vi "Test Switch when pressed.vi"(11 "Error in":errorcluster) -> (15 "Error out":errorcluster)   [LabVIEW 2020, in "Mechanical Actions Tests.lvlib"]
doc: "This VI is used to test the switch when pressed function"
uses:
  Mechanical Actions Tests.lvlib
  <vilib>/addons/_JKI Toolkits/Caraya/classes/Test Suite/Define Test Suite (JUnit Report).vi
  <vilib>/SLL Drona/APIs/Stimulus/ControlValue/SetValueAuto.vi
  <vilib>/SLL Drona/APIs/Assert/AssertControlValue/Greater.vi
  <vilib>/SLL Drona/APIs/Assert/AssertControlValue/Equal.vi
  <vilib>/SLL Drona/APIs/Stimulus/VI/CloseVI.vi
  <vilib>/Utility/error.llb/Error Cluster From Error Code.vi
  <vilib>/ErrorRing/Error Ring.xnode
  <vilib>/addons/_JKI Toolkits/Caraya/classes/Test Suite/Test Suite.lvclass
  <vilib>/addons/_JKI Toolkits/Caraya/classes/Test/Test.lvclass
  <vilib>/SLL Drona/Drona.lvlib
  <vilib>/SLL Drona/APIs/Stimulus/ControlValue/ControlValue.lvlib
  <vilib>/SLL Drona/APIs/Assert/AssertControlValue/AssertControlValue.lvlib
  <vilib>/Wiresmith Technology/G CLI/CLI Class/CLI.lvclass
  <vilib>/SLL Drona/APIs/Stimulus/VI/VI.lvlib
panel:
  # "SWITCH WHEN PRESSED TEST"
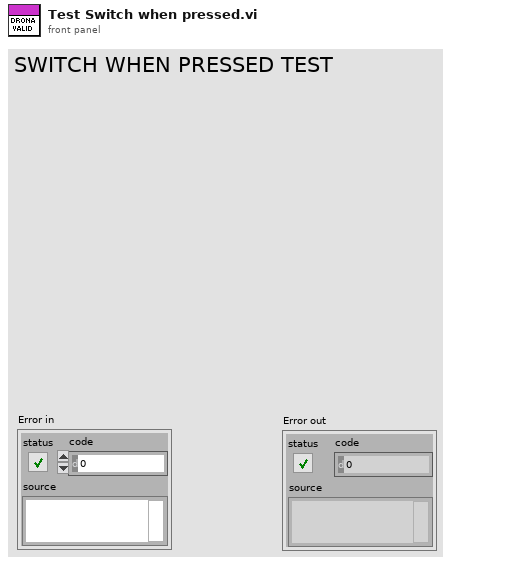
[diagram p1: front panel]
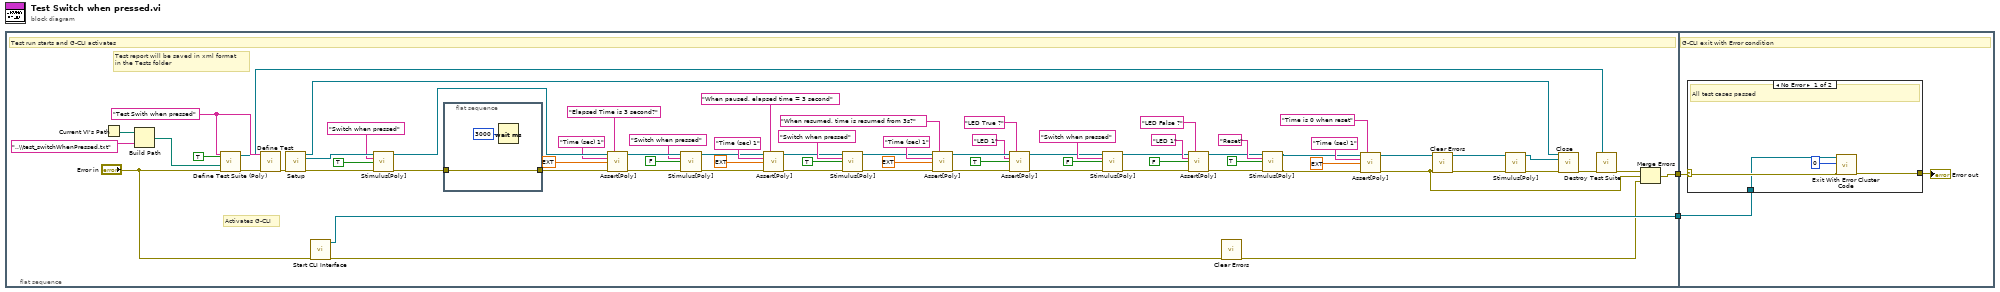
[diagram p0: block diagram]
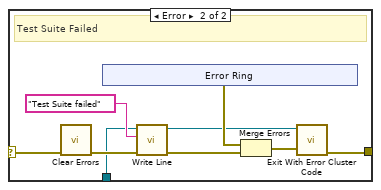
[diagram p2: hidden frame]
diagram:
  n1 = flat-sequence {
    tunnel: [w8] -> w2
    tunnel: [w6] -> w1
    tunnel: w2 -> [w78]
    tunnel: w1 -> [w77]
    frame #0 {
      w17 = "Test Swith when pressed" ("Label (VI Title)")
      # "Activates G-CLI"
      # "Test report will be saved in xml format\nin the Tests folder"
      # "Test run starts and G-CLI activates"
      n2 = Current VI's Path() -> (path=w15:path)
      n3 = Build Path(base path=w15, name or relative path="..\\test_switchWhenPressed.txt") -> (appended path=w13:path)
      n4 = call-poly <vilib>:"Define Test Suite (Poly).vi"("error in (no error)"="Error in", "Report Path"=w13, "Interactive"=TRUE, "Label (VI Title)"=w17) -> ("error out"=w18:errorcluster, "Test Suite"=w5:refnum<class "Test Suite.lvclass">)  [unwired: 5 in, 1 out]
      n5 = call <vilib>:"Define Test.vi"("error in (no error)"=w18, "Label (VI Title)"=w17) -> ("error out"=w74:errorcluster)  [unwired: 8 in, 1 out]
      n6 = call <vilib>:"Setup.vi"("error in"=w74) -> ("Application Ref"=w40:refnum<vi>, "VI Reference Out"=w72:refnum<vi>, "error out"=w73:errorcluster)  [unwired: 12 in]
      n7 = call <vilib>:"Start CLI Interface.vi"("error in (no error)"="Error in") -> ("error out"=w9:errorcluster, "CLI out"=w8:refnum<class "CLI.lvclass">)  [unwired: 7 in, 2 out]
      n8 = call-poly <vilib>:"Stimulus[Poly].vi"("VI Reference In"=w72, "Control Path"="Switch when pressed", "Value (Signaling)"=TRUE, "error in"=w73) -> ("VI Reference Out"=w67:refnum<vi>, "error out"=w69:errorcluster)  [unwired: 10 in]
      n9 = flat-sequence {
        tunnel: w69 -> [w76]
        tunnel: [w76] -> w68
        frame #0 {
          n10 = Wait (ms)(milliseconds to wait=u32 3000) -> ()  [unwired: 1 out]
        }
      }
      n11 = call-poly <vilib>:"Assert[Poly].vi"("VI Reference In"=w67, "Test Label"="Elapsed Time is 3 second?" ("Label"), "Control Path"="Time (sec) 1", "Control Value"=ext 3.0, "Error In"=w68) -> ("VI Reference Out"=w63:refnum<vi>, "Error Out"=w64:errorcluster)  [unwired: 9 in]
      n12 = call-poly <vilib>:"Stimulus[Poly].vi"("VI Reference In"=w63, "Control Path"="Switch when pressed", "Value (Signaling)"=FALSE, "error in"=w64) -> ("VI Reference Out"=w58:refnum<vi>, "error out"=w59:errorcluster)  [unwired: 10 in]
      n13 = call-poly <vilib>:"Assert[Poly].vi"("VI Reference In"=w58, "Test Label"="When paused, elapsed time = 3 second" ("Label"), "Control Path"="Time (sec) 1", "Control Value"=ext 3.0, "Error In"=w59) -> ("VI Reference Out"=w51:refnum<vi>, "Error Out"=w52:errorcluster)  [unwired: 9 in]
      n14 = call-poly <vilib>:"Stimulus[Poly].vi"("VI Reference In"=w51, "Control Path"="Switch when pressed", "Value (Signaling)"=TRUE, "error in"=w52) -> ("VI Reference Out"=w47:refnum<vi>, "error out"=w48:errorcluster)  [unwired: 10 in]
      n15 = call-poly <vilib>:"Assert[Poly].vi"("VI Reference In"=w47, "Test Label"="When resumed, time is resumed from 3s?" ("Label"), "Control Path"="Time (sec) 1", "Control Value"=ext 3.0, "Error In"=w48) -> ("VI Reference Out"=w36:refnum<vi>, "Error Out"=w33:errorcluster)  [unwired: 9 in]
      n16 = call-poly <vilib>:"Assert[Poly].vi"("VI Reference In"=w36, "Test Label"="LED True ?" ("Label"), "Control Path"="LED 1", "Control Value"=TRUE, "Error In"=w33) -> ("VI Reference Out"=w31:refnum<vi>, "Error Out"=w32:errorcluster)  [unwired: 9 in]
      n17 = call-poly <vilib>:"Stimulus[Poly].vi"("VI Reference In"=w31, "Control Path"="Switch when pressed", "Value (Signaling)"=FALSE, "error in"=w32) -> ("VI Reference Out"=w25:refnum<vi>, "error out"=w26:errorcluster)  [unwired: 10 in]
      n18 = call-poly <vilib>:"Assert[Poly].vi"("VI Reference In"=w25, "Test Label"="LED False ?" ("Label"), "Control Path"="LED 1", "Control Value"=FALSE, "Error In"=w26) -> ("VI Reference Out"=w24:refnum<vi>, "Error Out"=w23:errorcluster)  [unwired: 9 in]
      n19 = call <vilib>:"Clear Errors.vi"("error in (no error)"=w9) -> ("error out"=w7:errorcluster)  [unwired: 5 in, 1 out]
      n20 = call-poly <vilib>:"Stimulus[Poly].vi"("VI Reference In"=w24, "Control Path"="Reset", "Value (Signaling)"=TRUE, "error in"=w23) -> ("VI Reference Out"=w43:refnum<vi>, "error out"=w44:errorcluster)  [unwired: 10 in]
      n21 = call-poly <vilib>:"Assert[Poly].vi"("VI Reference In"=w43, "Test Label"="Time is 0 when reset" ("Label"), "Control Path"="Time (sec) 1", "Control Value"=ext 0.0, "Error In"=w44) -> ("VI Reference Out"=w21:refnum<vi>, "Error Out"=w3:errorcluster)  [unwired: 9 in]
      n22 = call <vilib>:"Clear Errors.vi"("error in (no error)"=w3) -> ("error out"=w4:errorcluster)  [unwired: 5 in, 1 out]
      n23 = call-poly <vilib>:"Stimulus[Poly].vi"("VI Reference In"=w21, "error in"=w4) -> ("VI Reference Out"=w20:refnum<vi>, "error out"=w19:errorcluster)  [unwired: 12 in]
      n24 = call <vilib>:"Close.vi"("Application Ref"=w40, "VI Reference"=w20, "error in"=w19) -> ("error out"=w11:errorcluster)  [unwired: 12 in]
      n25 = call-dynamic "Destroy Test Suite.vi"("error in (no error)"=w11, "Test Suite in"=w5) -> ("error out"=w10:errorcluster)  [unwired: 8 in, 1 out]
      n26 = Merge Errors(w10, w3, w7) -> (w6:errorcluster)
    }
    frame #1 {
      # "G-CLI exit with Error condition"
      n27 = case shown="No Error" w77 {
        selector: w77 -> [w83 w90]
        tunnel: [w82 w92] -> w79
        tunnel: w78 -> [w80 w85]
        frame No Error {
          # "All test cases passed"
          n28 = call <vilib>:"Exit With Error Cluster Code.vi"("error in (no error)"=w83, "No Error Code (0)"=0, "CLI in"=w80) -> ("error out"=w82:errorcluster)  [unwired: 8 in]
        }
        frame Error {
          # "Test Suite Failed"
          n29 = call <vilib>:"Clear Errors.vi"("error in (no error)"=w90) -> ("error out"=w89:errorcluster)  [unwired: 5 in, 1 out]
          n30 = xnode "Error Ring"() -> ("error out"=w87:errorcluster)
          n31 = call <vilib>:"Write Line.vi"("error in (no error)"=w89, "Text to Write"="Test Suite failed", "CLI in"=w85) -> ("error out"=w86:errorcluster, "CLI out"=w84:refnum<class "CLI.lvclass">)  [unwired: 7 in]
          n32 = Merge Errors(w87, w86) -> (w88:errorcluster)
          n33 = call <vilib>:"Exit With Error Cluster Code.vi"("error in (no error)"=w88, "CLI in"=w84) -> ("error out"=w92:errorcluster)  [unwired: 9 in]
        }
      }
      "Error out" <- w79
    }
  }
